vi "AddOrder.vi"(11 "buffer.in":u64[](array[numeric])=[2459274161843883858, 5279397646710161952, 5620492615227034656, 281474976710656, 0, 0, 0, 0, 0] format="%.0x") -> (3 "OrderBook.Command":T1={"type"=enum."AddOrder", "side"=66, "orderId "=3544385890602799695, "quantity"=20000, "symbol"=138719281473, "price"=1, "executed.qty"=0, "canceled.qty"=0, "remaining.qty"=0, "seconds"=0, "nanoseconds"=447000, "Add"=FALSE, "Edit"=FALSE, "Remove"=FALSE, "seq no"=0, "recv.time"=0, "parse.time"=0} {"symbol" format="%.0x"})   [LabVIEW 2020]
uses:
  Market.Data.Common/fpga/orderbook.command.type.ctl
  Market.Data.Common/fpga/fpganow.common.fpga.lvlib
  Market.Data.Common/fpga/orderbook.command.ctl
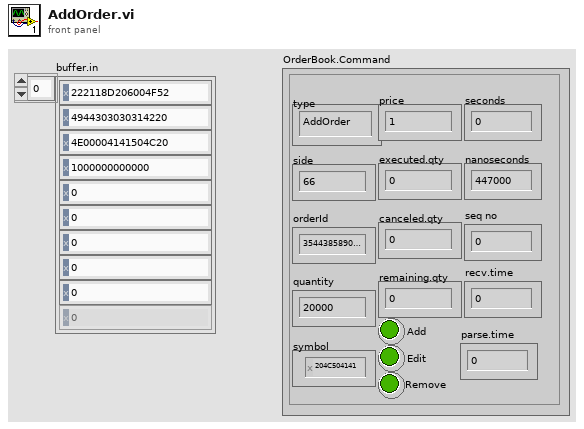
[diagram p1: front panel]
types:
  T1 = typedef "fpganow.common.fpga.lvlib/orderbook.command.ctl" = cluster{"type":T2, "side":u8, "orderId ":u64, "quantity":u32, "symbol":u64, "price":u64, "executed.qty":u32, "canceled.qty":u32, "remaining.qty":u32, "seconds":u64, "nanoseconds":u64, "Add":bool, "Edit":bool, "Remove":bool, "seq no":u32, "recv.time":u64, "parse.time":u64}
  T2 = typedef "fpganow.common.fpga.lvlib/orderbook.command.type.ctl" = enum8{"Time", "AddOrder", "OrderExecuted", "OrderExecutedAtPrice", "ReduceSize", "ModifyOrder", "DeleteOrder", "Get.Everything", "Get.All.Orders", "Get.Top"}
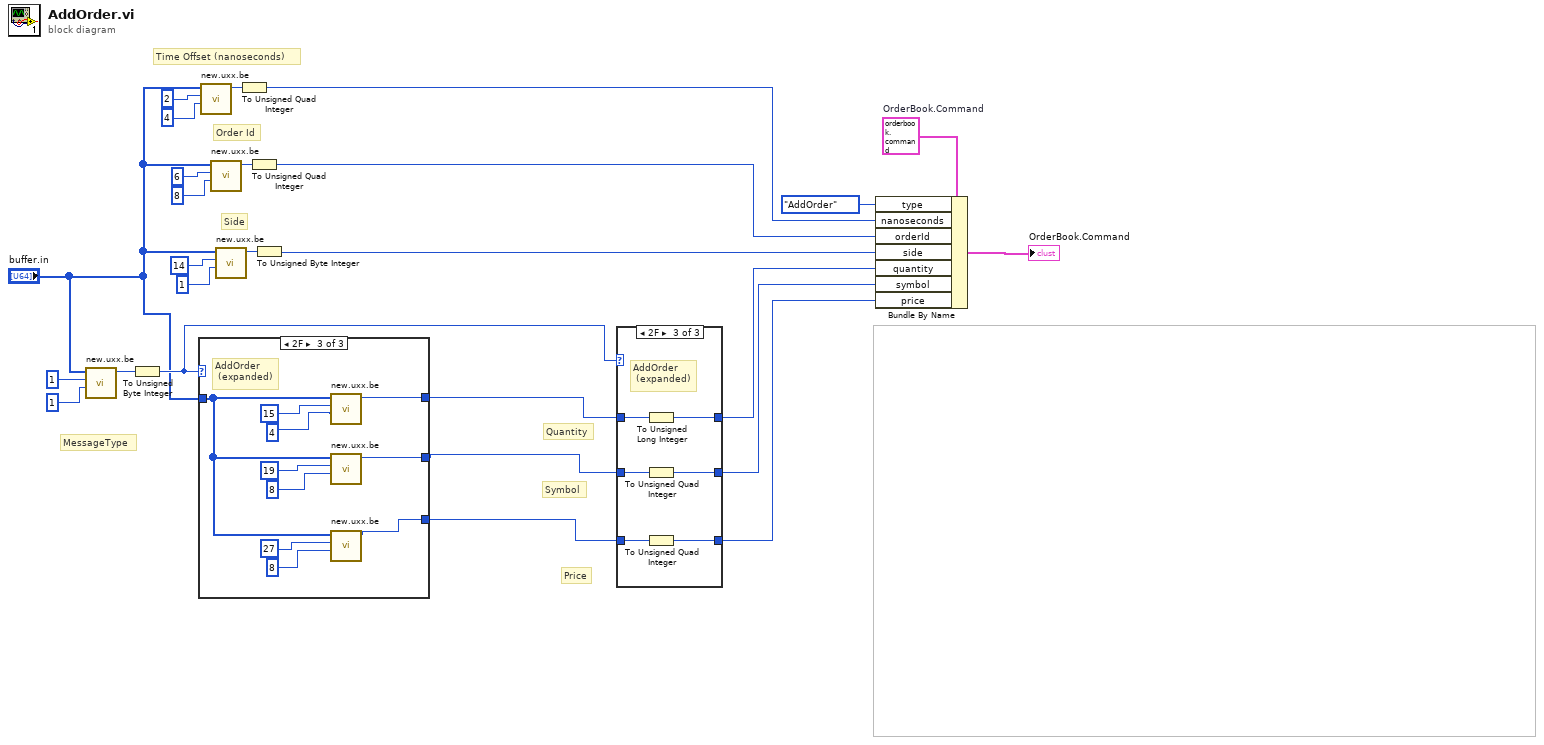
[diagram p0: block diagram]
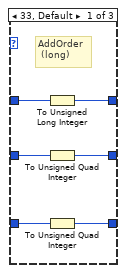
[diagram p2: hidden frame]
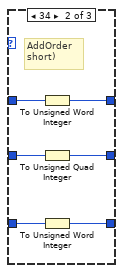
[diagram p3: hidden frame]
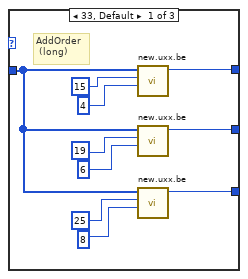
[diagram p4: hidden frame]
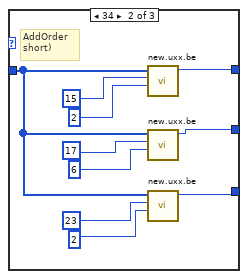
[diagram p5: hidden frame]
diagram:
  w23 = T1 {"type"=enum."AddOrder", "side"=0, "orderId "=0, "quantity"=0, "symbol"=0, "price"=0, "executed.qty"=0, "canceled.qty"=0, "remaining.qty"=0, "seconds"=0, "nanoseconds"=0, "Add"=FALSE, "Edit"=FALSE, "Remove"=FALSE, "seq no"=0, "recv.time"=0, "parse.time"=0}  # OrderBook.Command
  # "Price"
  # "Symbol"
  # "Quantity"
  # "Side"
  # "Order Id"
  # "Time Offset (nanoseconds)"
  # "MessageType"
  n1 = call "new.uxx.be.vi"("buffer (U64)"="buffer.in", "Start.Idx"=u8 1, "Length"=u8 1) -> ("Out.Value U64"=w24:u64)  [unwired: 7 in]
  n2 = To Unsigned Byte Integer(number=w24) -> (unsigned 8bit integer=w8:u8)
  n3 = case shown="2F" w8 {
    tunnel: "buffer.in" -> [w33 w46 w56]
    tunnel: [w34 w43 w55] -> w1
    tunnel: [w28 w37 w53] -> w3
    tunnel: [w27 w38 w54] -> w2
    frame 33, Default {
      # "AddOrder\n (long)"
      n4 = call "new.uxx.be.vi"("buffer (U64)"=w33, "Start.Idx"=u8 15, "Length"=u8 4) -> ("Out.Value U64"=w34:u64)  [unwired: 7 in]
      n5 = call "new.uxx.be.vi"("buffer (U64)"=w33, "Start.Idx"=u8 19, "Length"=u8 6) -> ("Out.Value U64"=w27:u64)  [unwired: 7 in]
      n6 = call "new.uxx.be.vi"("buffer (U64)"=w33, "Start.Idx"=u8 25, "Length"=u8 8) -> ("Out.Value U64"=w28:u64)  [unwired: 7 in]
    }
    frame 34 {
      # "AddOrder \nshort)"
      n7 = call "new.uxx.be.vi"("buffer (U64)"=w46, "Start.Idx"=u8 15, "Length"=u8 2) -> ("Out.Value U64"=w43:u64)  [unwired: 7 in]
      n8 = call "new.uxx.be.vi"("buffer (U64)"=w46, "Start.Idx"=u8 17, "Length"=u8 6) -> ("Out.Value U64"=w38:u64)  [unwired: 7 in]
      n9 = call "new.uxx.be.vi"("buffer (U64)"=w46, "Start.Idx"=u8 23, "Length"=u8 2) -> ("Out.Value U64"=w37:u64)  [unwired: 7 in]
    }
    frame 47 {
      # "AddOrder\n (expanded)"
      n10 = call "new.uxx.be.vi"("buffer (U64)"=w56, "Start.Idx"=u8 15, "Length"=u8 4) -> ("Out.Value U64"=w55:u64)  [unwired: 7 in]
      n11 = call "new.uxx.be.vi"("buffer (U64)"=w56, "Start.Idx"=u8 19, "Length"=u8 8) -> ("Out.Value U64"=w54:u64)  [unwired: 7 in]
      n12 = call "new.uxx.be.vi"("buffer (U64)"=w56, "Start.Idx"=u8 27, "Length"=u8 8) -> ("Out.Value U64"=w53:u64)  [unwired: 7 in]
    }
  }
  n13 = call "new.uxx.be.vi"("buffer (U64)"="buffer.in", "Start.Idx"=u8 2, "Length"=u8 4) -> ("Out.Value U64"=w18:u64)  [unwired: 7 in]
  n14 = call "new.uxx.be.vi"("buffer (U64)"="buffer.in", "Start.Idx"=u8 6, "Length"=u8 8) -> ("Out.Value U64"=w15:u64)  [unwired: 7 in]
  n15 = call "new.uxx.be.vi"("buffer (U64)"="buffer.in", "Start.Idx"=u8 14, "Length"=u8 1) -> ("Out.Value U64"=w12:u64)  [unwired: 7 in]
  n16 = To Unsigned Quad Integer(1:w18) -> (0:w11:u64)
  n17 = To Unsigned Quad Integer(1:w15) -> (0:w10:u64)
  n18 = To Unsigned Byte Integer(number=w12) -> (unsigned 8bit integer=w9:u8)
  n19 = case shown="2F" w8 {
    tunnel: [w59 w65 w71] -> w7
    tunnel: [w58 w64 w70] -> w6
    tunnel: [w57 w63 w69] -> w5
    tunnel: w1 -> [w62 w66 w73]
    tunnel: w3 -> [w60 w68 w74]
    tunnel: w2 -> [w61 w67 w72]
    frame 33, Default {
      # "AddOrder\n (long)"
      n20 = To Unsigned Long Integer(number=w62) -> (unsigned 32bit integer=w59:u32)
      n21 = To Unsigned Quad Integer(1:w61) -> (0:w58:u64)
      n22 = To Unsigned Quad Integer(1:w60) -> (0:w57:u64)
    }
    frame 34 {
      # "AddOrder \nshort)"
      n23 = To Unsigned Word Integer(number=w66) -> (unsigned 16bit integer=w65:u16)
      n24 = To Unsigned Quad Integer(1:w67) -> (0:w64:u64)
      n25 = To Unsigned Word Integer(number=w68) -> (unsigned 16bit integer=w63:u16)
    }
    frame 47 {
      # "AddOrder\n (expanded)"
      n26 = To Unsigned Long Integer(number=w73) -> (unsigned 32bit integer=w71:u32)
      n27 = To Unsigned Quad Integer(1:w72) -> (0:w70:u64)
      n28 = To Unsigned Quad Integer(1:w74) -> (0:w69:u64)
    }
  }
  n29 = Bundle By Name(cluster=w23, "type"=orderbook.command.type."AddOrder" ("OrderBook Command"), "nanoseconds"=w11, "orderId"=w10, "side"=w9, "quantity"=w7, "symbol"=w6, "price"=w5) -> (→"OrderBook.Command":T1)
